vi "Polarizer_calib_find_zero_6.vi"(2 "Tolerance":dbl=0.1, 3 "Find Zero":bool, 6 "Medir pasos\n por vuelta":bool, 7 "Angulo \ndeseado":dbl, 8 "Argumento":string="50", 9 "Número de motor":string="1", 10 "Pasos por \nvuelta":dbl=757.0, 11 "Go to angle":bool) -> ()   [LabVIEW 2013]
uses:
  <vilib>/Analysis/baseanly.llb/Mean (DBL).vi
  <vilib>/Utility/file.llb/Write To Spreadsheet File (DBL).vi
  <vilib>/regexp/Match Regular Expression.xnode
  <vilib>/Analysis/NI_AALBase.lvlib
panel:
  out "Find Zero S2":bool
  out "Error":dbl format="%#_4g"
  out "Min value":dbl
  out "Cero absoluto":dbl
  in  "Find Zero 2":bool
  in  "Pasos por vuelta para cada motor\nM1(757)        M2(661)      M3(744)      M4(751)":dbl[](array[numeric])=[757.0, 661.0, 744.0, 751.0]
  out "Angulo \nfinal":dbl
  out "Angulo por\npaso":dbl
  in  "Restart \n Arduino":bool
  in  "Stop VI":bool
  in  "wait until completion? (T)":bool=TRUE
  in  "Boolean 2":bool
  in  "Set speed":bool
  in  "Current Step":bool
  in  "Set Zero":bool
  in  "Shutter off":bool
  in  "Shutter on":bool
  in  "Stop":bool
  in  "Go to step":bool
  in  "Constant speed":bool
  in  "Comando":string
  in  "x":bool
  out "x > y?":bool
  in  "x1":bool
  out "Array":string[](array[string])
  in  "Tab Control":enum32{"Live Picture", "ICImagingControl "}(tab)
  out "Live Picture":picture
  in  "ICImagingControl 2":refnum<k7>(container)
  out "nearest integer value":dbl
  out "Terminal output":string
  in  "Directorio scripts ArduinoStepper.py":path=path "C:/Users/franjas/Documents/rutinas-calibracion-slm"
  out "Comando que está siendo enviado a python":string
  in  "Zero_bol":bool
  out "Current Value":dbl format="%0.2f"
  in  "Save history data":bool
  out "Waveform Chart":dbl(graph)
  out "Found minimum":bool=TRUE
  out "i old":i32
  out "Waveform Chart 2":dbl(graph)
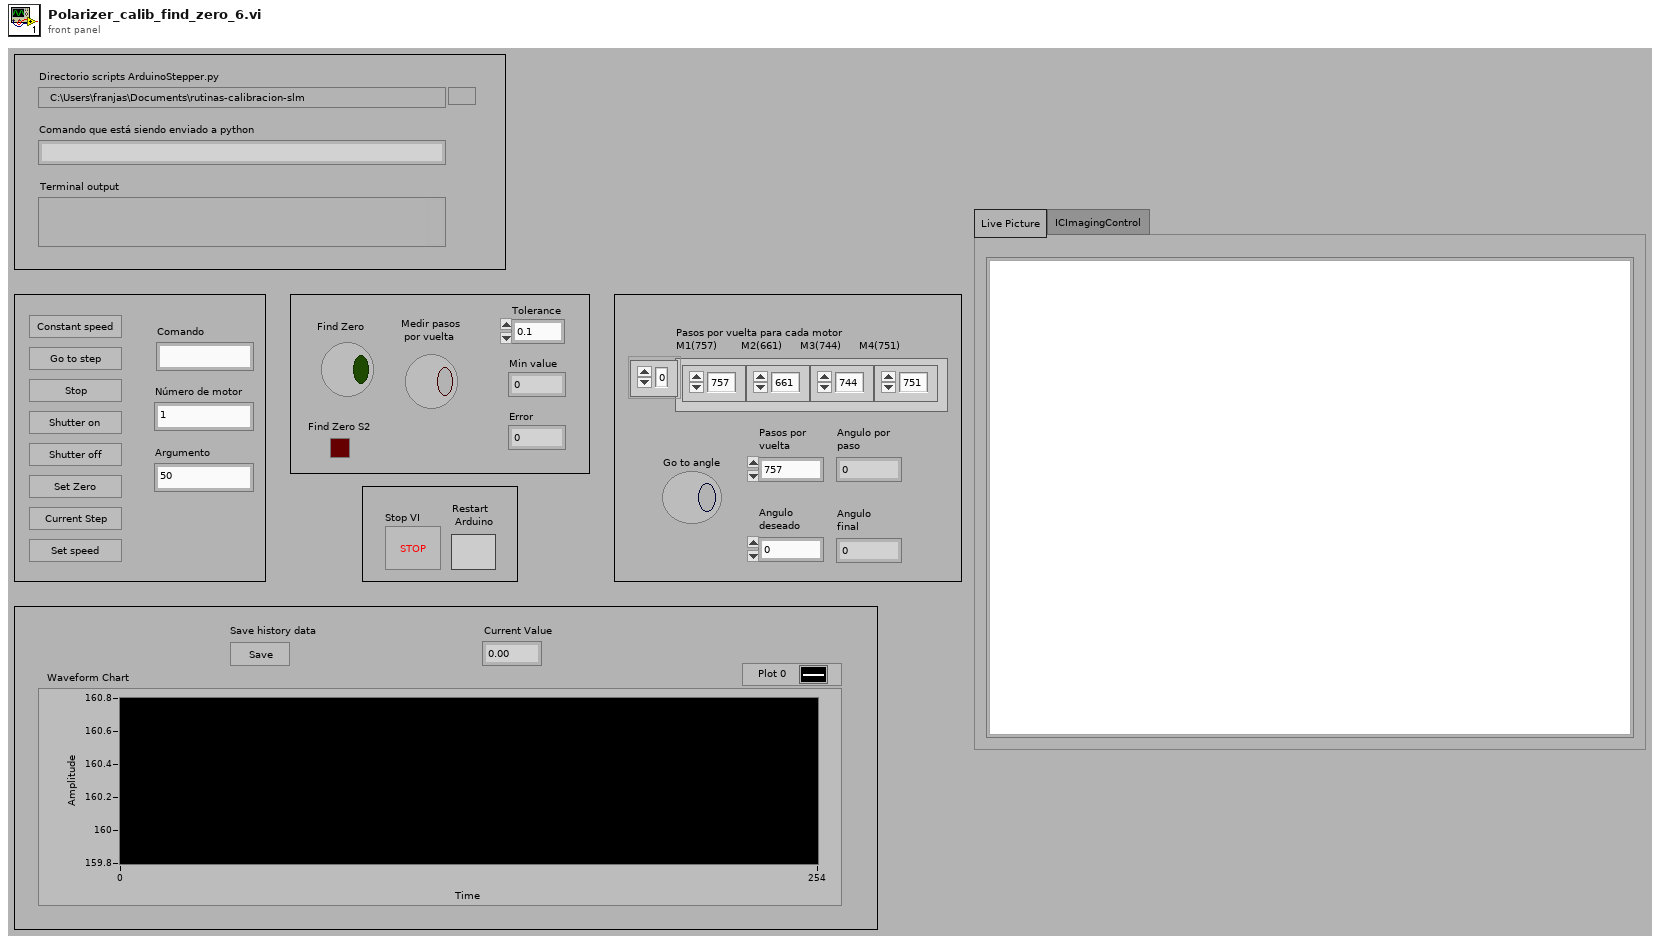
[diagram p1: front panel]
types:
  T1 = typedef "imagedata.ctl" = cluster{"image type":i32, "image depth":i32, "image":u8[], "mask":u8[], "colors":u32[], "Rectangle":cluster{"left":i16, "top":i16, "right":i16, "bottom":i16}}
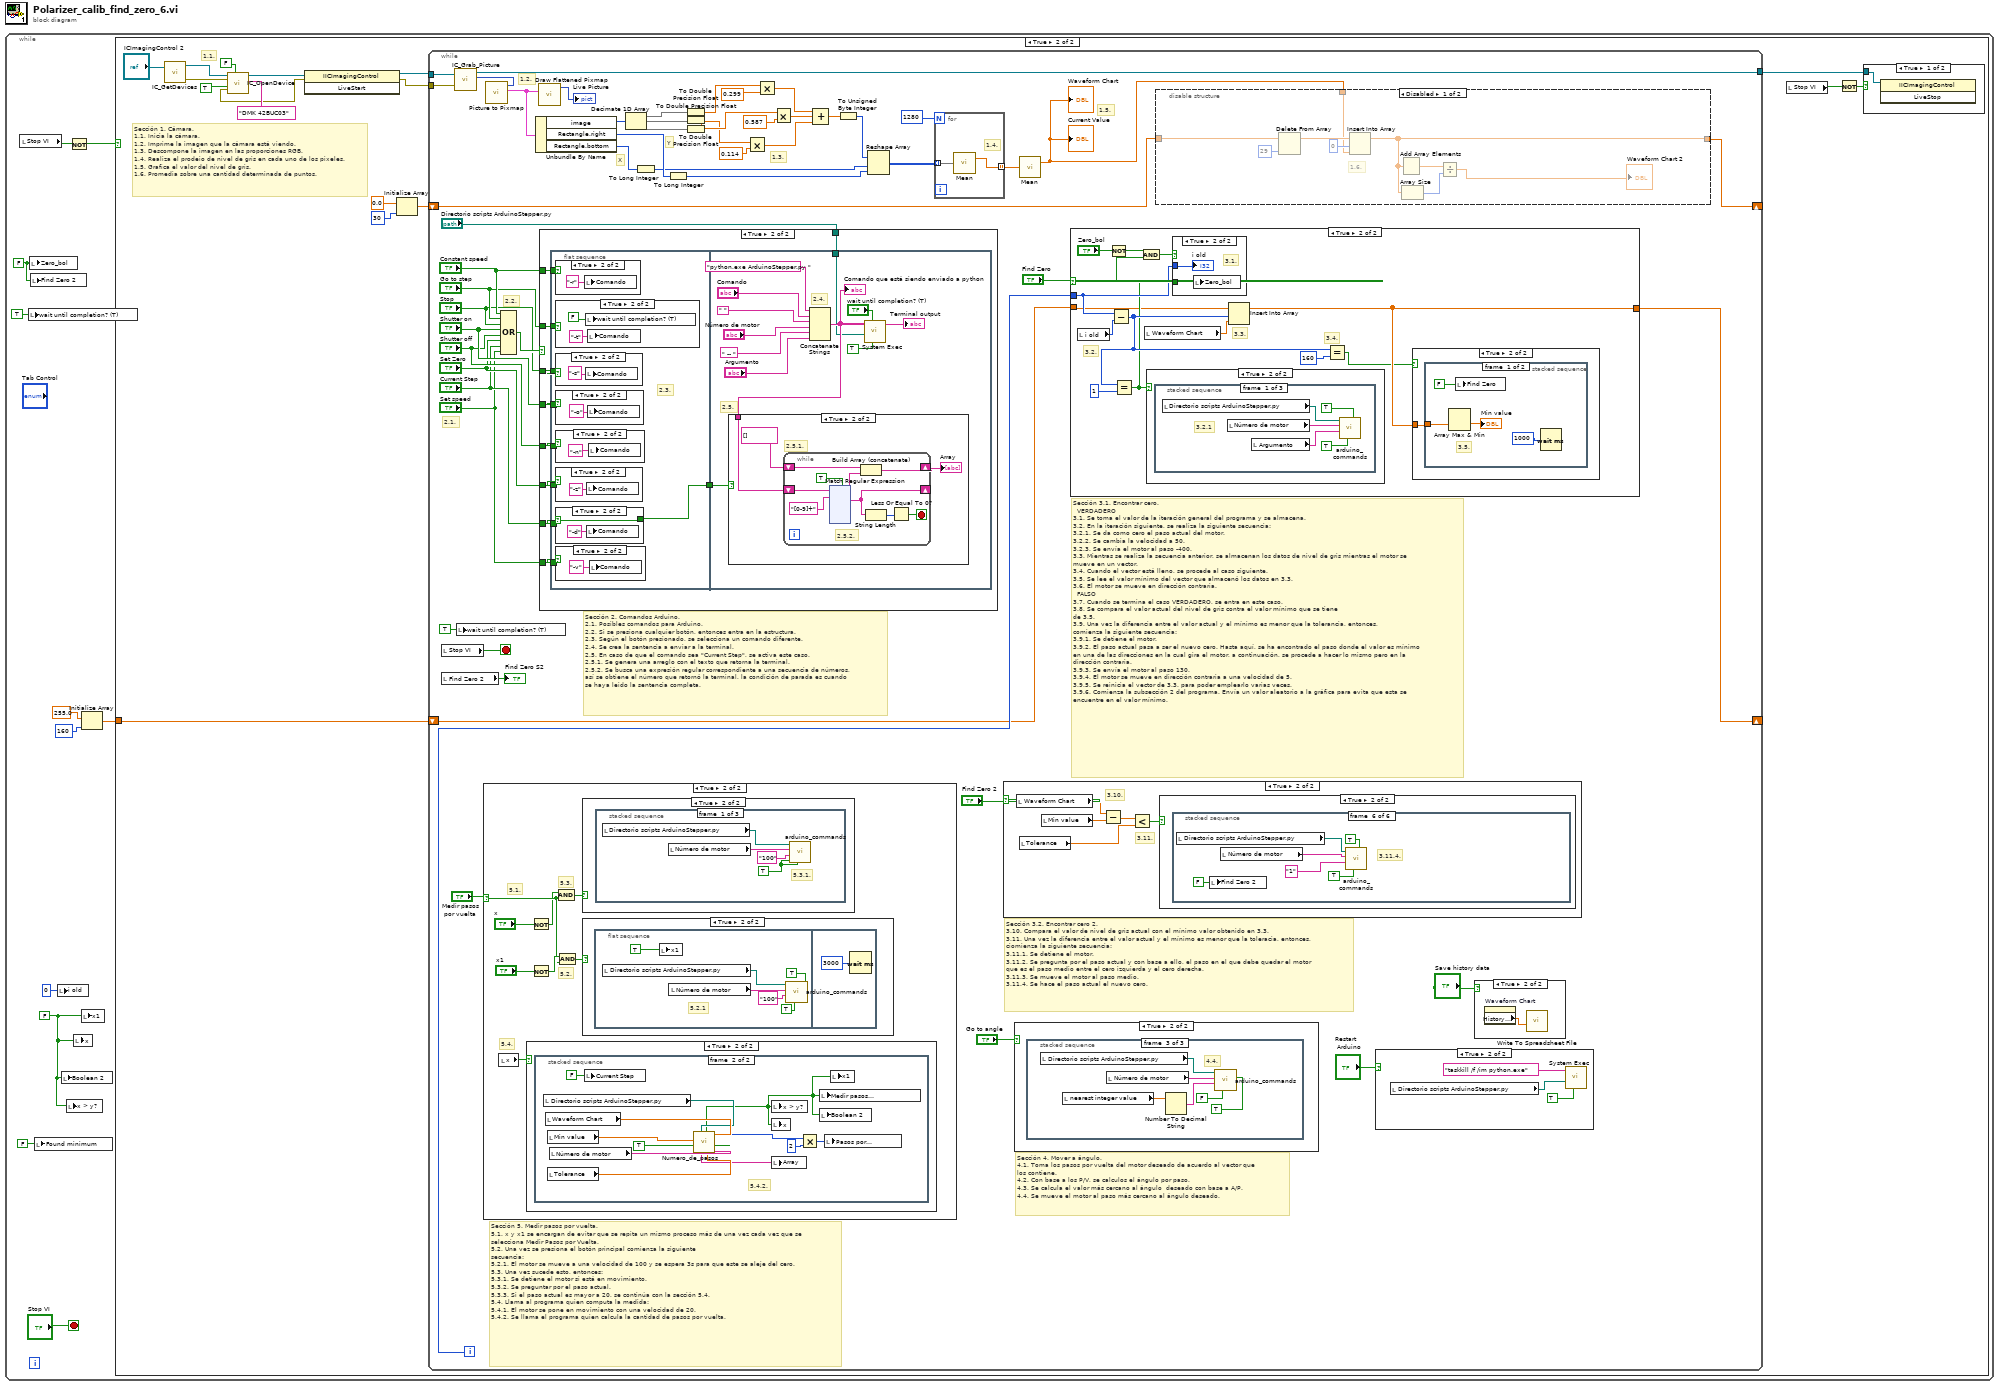
[diagram p0: block diagram]
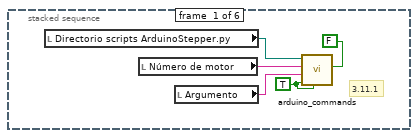
[diagram p6: hidden frame]
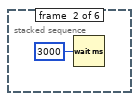
[diagram p7: hidden frame]
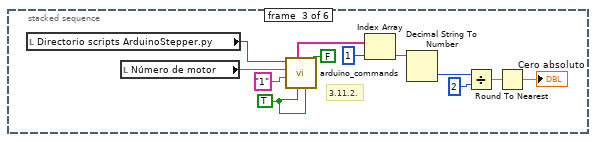
[diagram p8: hidden frame]
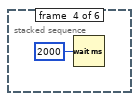
[diagram p9: hidden frame]
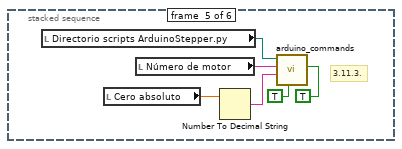
[diagram p10: hidden frame]
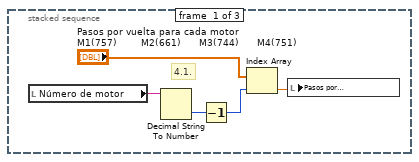
[diagram p13: hidden frame]
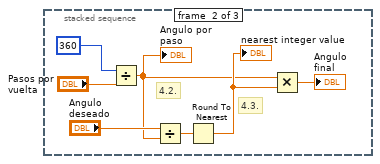
[diagram p14: hidden frame]
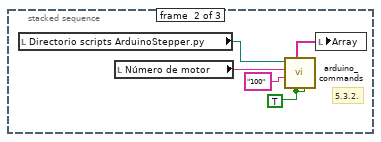
[diagram p17: hidden frame]
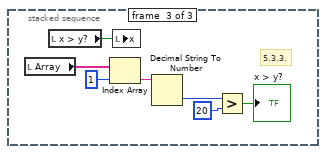
[diagram p18: hidden frame]
diagram:
  n1 = while {
    stop <- "Stop VI" stop-if-true
    w3 = FALSE ("Boolean")
    w1 = FALSE ("Zero_bol")
    n2 = local read "Stop VI"() -> (w5:bool)
    n3 = local write "wait until completion? (T)"(TRUE ("wait until completion? (T)")) -> ()
    n4 = local write "Zero_bol"(w1) -> ()
    n5 = local write "Find Zero 2"(w1) -> ()
    n6 = local write "Found minimum"(FALSE ("Found minimum")) -> ()
    n7 = local write "i old"(0 ("i old")) -> ()
    n8 = local write "Boolean 2"(w3) -> ()
    n9 = local write "x > y?"(w3) -> ()
    n10 = Not(x=w5) -> (.not. x?=w6:bool)
    n11 = local write "x"(w3) -> ()
    n12 = Initialize Array(255.0 ("element"), 160 ("dimension size")) -> (w9:dbl[])
    n13 = local write "x1"(w3) -> ()
    n14 = case shown="True" w6 {
      tunnel: w9 -> [_ w16]
      frame False {
      }
      frame True {
        # "Sección 1. Cámara. \n1.1. Inicia la cámara.\n1.2. Imprime la imagen que la cámara está viendo.\n1.3. Descompone la imagen en las proporciones RGB.\n1.4. Realiza el prodeio de nivel de gris en cada uno de los pixeles.\n1.5. Grafica el valor del nivel de gris.\n1.6. Promedia sobre una cantidad determinada de puntos."
        # "1.1."
        n15 = call <userlib>:"IC_GetDevices.vi"("ICImagingControl In"="ICImagingControl 2") -> ("ICImagingControl Out"=w26:refnum<k7>, "Error Out"=w22:errorcluster)  [unwired: 1 in, 1 out]
        n16 = call <userlib>:"IC_OpenDevice.vi"("Color"=FALSE, "Error In (no error)"=w22, "Live"=TRUE, "Device"="DMK 42BUC03", "ICImagingControl In"=w26) -> ("ICImagingControl Out"=w23:refnum<k7>, "Error Out"=w21:errorcluster)  [unwired: 1 in, 4 out]
        n17 = invoke class="IICImagingControl" method="LiveStart"(reference=w23, error in=w21) -> (reference out=w15:refnum<k7>, error out=w20:errorcluster)  [unwired: 1 in, 1 out]
        n18 = Initialize Array "Initialize Array"(0.0 ("element"), 30 ("dimension size")) -> (w14:dbl[])
        n19 = while {
          tunnel: w15 -> [w78]
          tunnel: w20 -> [w48]
          tunnel: [w79] -> w19
          shift-right: [w29] -> _
          shift-left: w14 -> [w60]
          shift-right: [w30] -> _
          shift-left: w16 -> [w58]
          i -> [w59]
          stop <- w54 stop-if-true
          # "Sección 5. Medir pasos por vuelta.\n5.1. x y x1 se encargan de evitar que se repita un mismo proceso más de una vez cada vez que se \nselecciona Medir Pasos por Vuelta. \n5.2. Una vez se presiona el botón principal comienza la siguiente\nsecuencia:\n5.2.1. El motor se mueve a una velocidad de 100 y se espera 3s para que este se aleje del cero.\n5.3. Una vez sucede esto, entonces:\n5.3.1. Se detiene el motor si está en movimiento.\n5.3.2. Se preguntar por el paso actual.\n5.3.3. Si el paso actual es mayor a 20, se continúa con la sección 5.4.\n5.4. Llama al programa quien computa la medida:\n5.4.1. El motor se pone en movimiento con una velocidad de 20.\n5.4.2. Se llama el programa quien calcula la cantidad de pasos por vuelta."
          # "Sección 3.2. Encontrar cero 2.\n3.10. Compara el valor de nivel de gris actual con el mínimo valor obtenido en 3.3.\n3.11. Una vez la diferencia entre el valor actual y el mínimo es menor que la toleracia, entonces, \nciomienza la siguiente secuencia:\n3.11.1. Se detiene el motor.\n3.11.2. Se pregunta por el paso actual y con base a ello, el paso en el que debe quedar el motor\nque es el paso medio entre el cero izquierda y el cero derecha.\n3.11.3. Se mueve el motor al paso medio.\n3.11.4. Se hace el paso actual el nuevo cero."
          # "Sección 3.1. Encontrar cero.\n  VERDADERO\n3.1. Se toma el valor de la iteración general del programa y se almacena.\n3.2. En la iteración siguiente, se realiza la siguiente secuencia:\n3.2.1. Se da como cero el paso actual del motor.\n3.2.2. Se cambia la velocidad a 50.\n3.2.3. Se envía el motor al paso -400.\n3.3. Mientras se realiza la secuencia anterior, se almacenan los datos de nivel de gris mientras el motor se \nmueve en un vector.\n3.4. Cuando el vector está lleno, se procede al caso siguiente.\n3.5. Se lee el valor mínimo del vector que almacenó los datos en 3.3. \n3.6. El motor se mueve en dirección contraria.\n  FALSO\n3.7. Cuando se termina el caso VERDADERO, se entra en este caso.\n3.8. Se compara el valor actual del nivel de gris contra el valor mínimo que se tiene\nde 3.5.\n3.9. Una vez la diferencia entre el valor actual y el mínimo es menor que la tolerancia, entonces, \ncomienza la siguiente secuencia:\n3.9.1. Se detiene el motor.\n3.9.2. El paso actual pasa a ser el nuevo cero. Hasta aquí, se ha encontrado el paso donde el valor es mínimo\nen una de las direcciones en la cual gira el motor, a continuación, se procede a hacer lo mismo pero en la \ndirección contraria. \n3.9.3. Se envía el motor al paso 130.\n3.9.4. El motor se mueve en dirección contraria a una velocidad de 5.\n3.9.5. Se reinicia el vector de 3.3. para poder emplearlo varias veces.\n3.9.6. Comienza la subsección 2 del programa. Envía un valor aleatorio a la gráfica para evita que esta se \nencuentre en el valor mínimo."
          # "Sección 4. Mover a ángulo.\n4.1. Toma los pasos por vuelta del motor deseado de acuerdo al vector que\nlos contiene.\n4.2. Con base a los P/V, se calculos el ángulo por paso.\n4.3. Se calcula el valor más cercano al ángulo  deseado con base a A/P.\n4.4. Se mueve el motor al paso más cercano al ángulo deseado."
          # "2.2."
          # "2.1."
          # "Sección 2. Comandos Arduino.\n2.1. Posibles comandos para Arduino.\n2.2. Si se presiona cualquier botón, entonces entra en la estructura.\n2.3. Según el botón presionado, se selecciona un comando diferente.\n2.4. Se crea la sentencia a enviar a la terminal.\n2.5. En caso de que el comando sea \"Current Step\", se activa este caso.\n2.5.1. Se genera una arreglo con el texto que retorna la terminal.\n2.5.2. Se busca una expresión regular correspondiente a una secuencia de números,\nasí se obtiene el número que retornó la terminal, la condición de parada es cuando\nse haya leido la sentencia completa."
          # "1.5."
          # "1.3."
          # "1.2."
          # "Y"
          # "X"
          n20 = local read "Stop VI"() -> (w54:bool)
          n21 = local read "Find Zero 2"() -> (→"Find Zero S2":bool)
          n22 = call <userlib>:"IC_Grab_Picture.vi"("ICImagingControl In"=w78, "Error In (no error)"=w48) -> ("ICImagingControl Out"=w79:refnum<k7>, "Picture Out"=w81:picture)  [unwired: 2 out]
          n23 = local write "wait until completion? (T)"(TRUE ("wait until completion? (T)")) -> ()
          n24 = case shown="True" "Medir pasos\n por vuelta" {
            selector: "Medir pasos\n por vuelta" -> [_ w143]
            frame False {
            }
            frame True {
              # "5.4."
              # "5.3."
              # "5.2."
              # "5.1."
              n25 = local read "x"() -> (w140:bool)
              n26 = case shown="True" w140 {
                frame False {
                }
                frame True {
                  n27 = stacked-sequence {
                    frame #0 {
                      n28 = Not(x="Boolean 2") -> (.not. x?=w171:bool)
                      n29 = case shown="True" w171 {
                        frame False {
                        }
                        frame True {
                          w174 = TRUE ("Constant speed")
                          # "5.4.1."
                          n30 = local read "Directorio scripts ArduinoStepper.py"() -> (w176:path)
                          n31 = local read "Número de motor"() -> (w177:string)
                          n32 = local write "Boolean 2"(w174) -> ()
                          n33 = call "arduino_commands.vi"("Constant speed"=w174, "Wait until completion? (T)"=FALSE ("wait until completion? (T)"), "Argumento"="20", "Número de motor"=w177, "Directorio scripts ArduinoStepper.py"=w176) -> ()  [unwired: 6 in, 1 out]
                        }
                      }
                    }
                    frame #1 {
                      # "5.4.2."
                      n34 = local read "Directorio scripts ArduinoStepper.py"() -> (w187:path)
                      n35 = local read "Waveform Chart"() -> (w189:dbl)
                      n36 = local read "Min value"() -> (w188:dbl)
                      n37 = local read "Tolerance"() -> (w185:dbl)
                      n38 = local read "Número de motor"() -> (w186:string)
                      n39 = local write "Current Step"(FALSE ("Current Step")) -> ()
                      n40 = call "Numero_de_pasos.vi"("Tolerance"=w185, "Directorio scripts ArduinoStepper.py"=w187, "Número de motor"=w186, "Medir pasos por\nvuelta"=TRUE ("Medir pasos por\nvuelta"), "Minimo"=w188, "Valor actual"=w189) -> ("Media vuelta"=w182:i32, "Proceso en \nejecución"=w179:bool, "Array"=w178:string[])  [unwired: 3 in]
                      n41 = local write "x > y?"(w179) -> ()
                      n42 = local write "x"(w179) -> ()
                      n43 = local write "Array"(w178) -> ()
                      n44 = Multiply(x=w182, y=2) -> (x*y=w180:i32)
                      n45 = local write "Medir pasos\n por vuelta"(w179) -> ()
                      n46 = local write "Boolean 2"(w179) -> ()
                      n47 = local write "Pasos por \nvuelta"(w180) -> ()
                      n48 = local write "x1"(w179) -> ()
                    }
                  }
                }
              }
              n49 = Not(x="x") -> (.not. x?=w141:bool)
              n50 = Not(x="x1") -> (.not. x?=w147:bool)
              n51 = And(x=w141, y=w143) -> (x .and. y?=w144:bool)
              n52 = And(x=w147, y=w143) -> (x .and. y?=w145:bool)
              n53 = case shown="True" w144 {
                frame False {
                }
                frame True {
                  n54 = stacked-sequence {
                    frame #0 {
                      w148 = TRUE ("Constant speed")
                      # "5.3.1."
                      n55 = local read "Directorio scripts ArduinoStepper.py"() -> (w150:path)
                      n56 = local read "Número de motor"() -> (w151:string)
                      n57 = call "arduino_commands.vi"("Wait until completion? (T)"=w148, "Stop"=w148, "Argumento"="100", "Número de motor"=w151, "Directorio scripts ArduinoStepper.py"=w150) -> ()  [unwired: 6 in, 1 out]
                    }
                    frame #1 {
                      w152 = TRUE ("wait until completion? (T)")
                      # "5.3.2."
                      n58 = local read "Directorio scripts ArduinoStepper.py"() -> (w155:path)
                      n59 = local read "Número de motor"() -> (w156:string)
                      n60 = call "arduino_commands.vi"("Current Step"=w152, "Wait until completion? (T)"=w152, "Argumento"="100", "Número de motor"=w156, "Directorio scripts ArduinoStepper.py"=w155) -> ("Retorno terminal"=w153:string[])  [unwired: 6 in]
                      n61 = local write "Array"(w153) -> ()
                    }
                    frame #2 {
                      # "5.3.3."
                      n62 = local read "Array"() -> (w161:string[])
                      n63 = local read "x > y?"() -> (w159:bool)
                      n64 = Index Array(array=w161, index=1) -> (element=w160:string)
                      n65 = local write "x"(w159) -> ()
                      n66 = Decimal String To Number(string=w160) -> (number=w162:i32)  [unwired: 2 in, 1 out]
                      n67 = Greater?(x=w162, y=20) -> (0:→"x > y?":bool)
                    }
                  }
                }
              }
              n68 = case shown="True" w145 {
                frame False {
                }
                frame True {
                  n69 = flat-sequence {
                    frame #0 {
                      # "5.2.1"
                      n70 = local read "Directorio scripts ArduinoStepper.py"() -> (w168:path)
                      n71 = local write "x1"(TRUE ("Boolean")) -> ()
                      n72 = local read "Número de motor"() -> (w167:string)
                      n73 = call "arduino_commands.vi"("Constant speed"=TRUE, "Wait until completion? (T)"=TRUE ("wait until completion? (T)"), "Argumento"="100", "Número de motor"=w167, "Directorio scripts ArduinoStepper.py"=w168) -> ()  [unwired: 6 in, 1 out]
                    }
                    frame #1 {
                      n74 = Wait (ms)(milliseconds to wait=u32 3000) -> ()  [unwired: 1 out]
                    }
                  }
                }
              }
            }
          }
          n75 = call <vilib>:"Picture to Pixmap.vi"("picture"=w81) -> ("image data"=w71:T1)  [unwired: 9 in, 1 out]
          n76 = Compound Arithmetic op=OR("Constant speed", "Go to step", "Stop", "Shutter on", "Shutter off", "Set Zero", "Current Step", "Set speed") -> (w42:bool)
          n77 = Unbundle By Name(w71) -> ("image"=w47:u8[], "Rectangle.right"=w75:i16, "Rectangle.bottom"=w73:i16)
          n78 = call <vilib>:"Draw Flattened Pixmap.vi"("image data"=w71) -> ("new picture"=→"Live Picture":picture)  [unwired: 8 in]
          n79 = case shown="True" w42 {
            tunnel: "Constant speed" -> [_ w292]
            tunnel: "Go to step" -> [_ w291]
            tunnel: "Stop" -> [_ w290]
            tunnel: "Shutter on" -> [_ w289]
            tunnel: "Shutter off" -> [_ w288]
            tunnel: "Set Zero" -> [_ w287]
            tunnel: "Current Step" -> [_ w286]
            tunnel: "Set speed" -> [_ w285]
            tunnel: "Directorio scripts ArduinoStepper.py" -> [_ w283]
            frame False {
            }
            frame True {
              n80 = flat-sequence {
                tunnel: w292 -> [w301]
                tunnel: w291 -> [w300]
                tunnel: w290 -> [w299]
                tunnel: w289 -> [w298]
                tunnel: w288 -> [w297]
                tunnel: w287 -> [w296]
                tunnel: w286 -> [w295]
                tunnel: w285 -> [w294]
                tunnel: [w293] -> w284
                tunnel: w284 -> [w315]
                tunnel: w283 -> [w314]
                frame #0 {
                  # "2.3."
                  n81 = case shown="True" w301 {
                    frame False {
                    }
                    frame True {
                      n82 = local write "Comando"("-r" ("Comando")) -> ()
                    }
                  }
                  n83 = case shown="True" w300 {
                    frame False {
                    }
                    frame True {
                      n84 = local write "wait until completion? (T)"(FALSE ("wait until completion? (T)")) -> ()
                      n85 = local write "Comando"("-t" ("Comando")) -> ()
                    }
                  }
                  n86 = case shown="True" w299 {
                    frame False {
                    }
                    frame True {
                      n87 = local write "Comando"("-s" ("Comando")) -> ()
                    }
                  }
                  n88 = case shown="True" w298 {
                    frame False {
                    }
                    frame True {
                      n89 = local write "Comando"("-o" ("Comando")) -> ()
                    }
                  }
                  n90 = case shown="True" w297 {
                    frame False {
                    }
                    frame True {
                      n91 = local write "Comando"("-n" ("Comando")) -> ()
                    }
                  }
                  n92 = case shown="True" w296 {
                    frame False {
                    }
                    frame True {
                      n93 = local write "Comando"("-z" ("Comando")) -> ()
                    }
                  }
                  n94 = case shown="True" w295 {
                    selector: w295 -> [w303 w304]
                    tunnel: [w303 w304] -> w293
                    frame False {
                    }
                    frame True {
                      n95 = local write "Comando"("-d" ("Comando")) -> ()
                    }
                  }
                  n96 = case shown="True" w294 {
                    frame False {
                    }
                    frame True {
                      n97 = local write "Comando"("-v" ("Comando")) -> ()
                    }
                  }
                }
                frame #1 {
                  # "2.5."
                  # "2.4."
                  n98 = Concatenate Strings("python.exe ArduinoStepper.py ", "Comando", " " ("string"), "Número de motor", " -- ", "Argumento") -> (w317:string)
                  "Comando que está siendo enviado a python" <- w317
                  n99 = call <vilib>:"System Exec.vi"("run minimized? (F)"=TRUE, "wait until completion? (T)"="wait until completion? (T)", "working directory"=w314, "command line"=w317) -> ("standard output"=w324:string)  [unwired: 4 in, 3 out]
                  "Terminal output" <- w324
                  n100 = case shown="True" w315 {
                    tunnel: w324 -> [_ w327]
                    frame False {
                    }
                    frame True {
                      # "2.5.1."
                      n101 = while {
                        shift-right: [w335] -> _
                        shift-left: w327 -> [w329]
                        shift-right: [w333] -> w326
                        shift-left: string[] [] -> [w331]
                        stop <- w328 stop-if-true
                        # "2.5.2."
                        n102 = xnode "Match Regular Expression"("input string"=w329, "regular expression"="[0-9]+", "multiline? (F)"=TRUE) -> ("whole match"=w332:string, "after match"=w335:string)  [unwired: 3 in, 5 out]
                        n103 = Build Array (concatenate)(w331, w332) -> (w333:string[])
                        n104 = String Length(string=w335) -> (length=w334:i32)
                        n105 = Less Or Equal To 0?(x=w334) -> (x <= 0?=w328:bool)
                      }
                      "Array" <- w326
                    }
                  }
                }
              }
            }
          }
          n106 = Decimate 1D Array(w47) -> (w61:u8[], w46:u8[], w45:u8[])
          n107 = To Long Integer(number=w73) -> (32bit integer=w72:i32)
          n108 = To Long Integer(number=w75) -> (32bit integer=w74:i32)
          n109 = To Double Precision Float(number=w61) -> (double precision float=w69:dbl[])
          n110 = To Double Precision Float(number=w46) -> (double precision float=w68:dbl[])
          n111 = To Double Precision Float(number=w45) -> (double precision float=w67:dbl[])
          n112 = Multiply(x=w67, y=0.114) -> (x*y=w62:dbl[])
          n113 = Multiply(x=w69, y=0.299) -> (x*y=w64:dbl[])
          n114 = Multiply(x=w68, y=0.587) -> (x*y=w63:dbl[])
          n115 = Compound Arithmetic op=ADD(w64, w63, w62) -> (w43:dbl[])
          n116 = To Unsigned Byte Integer(number=w43) -> (unsigned 8bit integer=w76:u8[])
          n117 = Reshape Array(w76, w72, w74) -> (w70:u8[][])
          n118 = for {
            N: 1280 -> [_]
            tunnel: [w455] -> w80 mode=indexing
            tunnel: w70 -> [w454] mode=indexing
            # "1.4."
            n119 = call-poly <vilib>:"Mean.vi"("X"=w454) -> ("mean"=w455:dbl)  [unwired: 1 out]
          }
          n120 = case shown="True" "Find Zero 2" {
            frame False {
            }
            frame True {
              # "3.11."
              # "3.10."
              n121 = local read "Waveform Chart"() -> (w87:dbl)
              n122 = local read "Tolerance"() -> (w85:dbl)
              n123 = local read "Min value"() -> (w86:dbl)
              n124 = Subtract(x=w87, y=w86) -> (x-y=w84:dbl)
              n125 = Less?(x=w84, y=w85) -> (x < y?=w83:bool)
              n126 = case shown="True" w83 {
                frame False {
                }
                frame True {
                  n127 = stacked-sequence {
                    frame #0 {
                      w88 = TRUE ("Stop")
                      # "3.11.1"
                      n128 = local read "Directorio scripts ArduinoStepper.py"() -> (w90:path)
                      n129 = local read "Número de motor"() -> (w91:string)
                      n130 = local read "Argumento"() -> (w92:string)
                      n131 = call "arduino_commands.vi"("Go to step"=FALSE, "Wait until completion? (T)"=w88, "Stop"=w88, "Argumento"=w92, "Número de motor"=w91, "Directorio scripts ArduinoStepper.py"=w90) -> ()  [unwired: 5 in, 1 out]
                    }
                    frame #1 {
                      n132 = Wait (ms)(milliseconds to wait=u32 3000) -> ()  [unwired: 1 out]
                    }
                    frame #2 {
                      w101 = TRUE ("Constant speed")
                      # "3.11.2."
                      n133 = local read "Directorio scripts ArduinoStepper.py"() -> (w99:path)
                      n134 = local read "Número de motor"() -> (w100:string)
                      n135 = call "arduino_commands.vi"("Go to step"=FALSE, "Current Step"=w101, "Wait until completion? (T)"=w101, "Argumento"="1", "Número de motor"=w100, "Directorio scripts ArduinoStepper.py"=w99) -> ("Retorno terminal"=w104:string[])  [unwired: 5 in]
                      n136 = Index Array(array=w104, index=1) -> (element=w103:string)
                      n137 = Decimal String To Number(string=w103) -> (number=w97:i32)  [unwired: 2 in, 1 out]
                      n138 = Divide(x=w97, y=2) -> (x/y=w96:dbl)
                      n139 = Round To Nearest(number=w96) -> (nearest integer value=→"Cero absoluto":dbl)
                    }
                    frame #3 {
                      n140 = Wait (ms)(milliseconds to wait=u32 2000) -> ()  [unwired: 1 out]
                    }
                    frame #4 {
                      # "3.11.3."
                      n141 = local read "Directorio scripts ArduinoStepper.py"() -> (w110:path)
                      n142 = local read "Cero absoluto"() -> (w109:dbl)
                      n143 = local read "Número de motor"() -> (w111:string)
                      n144 = Number To Decimal String(number=w109) -> (decimal integer string=w112:string)  [unwired: 1 in]
                      n145 = call "arduino_commands.vi"("Go to step"=TRUE, "Wait until completion? (T)"=TRUE ("wait until completion? (T)"), "Argumento"=w112, "Número de motor"=w111, "Directorio scripts ArduinoStepper.py"=w110) -> ()  [unwired: 6 in, 1 out]
                    }
                    frame #5 {
                      # "3.11.4."
                      n146 = local read "Directorio scripts ArduinoStepper.py"() -> (w117:path)
                      n147 = local write "Find Zero 2"(FALSE ("Find Zero 2")) -> ()
                      n148 = local read "Número de motor"() -> (w116:string)
                      n149 = call "arduino_commands.vi"("Set zero"=TRUE, "Wait until completion? (T)"=TRUE, "Argumento"="1", "Número de motor"=w116, "Directorio scripts ArduinoStepper.py"=w117) -> ()  [unwired: 6 in, 1 out]
                    }
                  }
                }
              }
            }
          }
          n150 = case shown="True" "Go to angle" {
            frame False {
            }
            frame True {
              n151 = stacked-sequence {
                frame #0 {
                  # "4.1."
                  n152 = local read "Número de motor"() -> (w125:string)
                  n153 = Decimal String To Number(string=w125) -> (number=w126:i32)  [unwired: 2 in, 1 out]
                  n154 = Decrement(x=w126) -> (x-1=w123:i32)
                  n155 = Index Array(array="Pasos por vuelta para cada motor\nM1(757)        M2(661)      M3(744)      M4(751)", index=w123) -> (element=w124:dbl)
                  n156 = local write "Pasos por \nvuelta"(w124) -> ()
                }
                frame #1 {
                  # "4.3."
                  # "4.2."
                  n157 = Divide(x=360, y="Pasos por \nvuelta") -> (x/y=w128:dbl)
                  "Angulo por\npaso" <- w128
                  n158 = Divide(x="Angulo \ndeseado", y=w128) -> (x/y=w130:dbl)
                  n159 = Round To Nearest(number=w130) -> (nearest integer value=w129:dbl)
                  "nearest integer value" <- w129
                  n160 = Multiply(x=w128, y=w129) -> (x*y=→"Angulo \nfinal":dbl)
                }
                frame #2 {
                  # "4.4."
                  n161 = local read "Directorio scripts ArduinoStepper.py"() -> (w139:path)
                  n162 = local read "nearest integer value"() -> (w135:dbl)
                  n163 = local read "Número de motor"() -> (w138:string)
                  n164 = Number To Decimal String(number=w135) -> (decimal integer string=w136:string)  [unwired: 1 in]
                  n165 = call "arduino_commands.vi"("Go to step"=TRUE, "Wait until completion? (T)"=FALSE ("wait until completion? (T)"), "Argumento"=w136, "Número de motor"=w138, "Directorio scripts ArduinoStepper.py"=w139) -> ()  [unwired: 6 in, 1 out]
                }
              }
            }
          }
          n166 = call-poly <vilib>:"Mean.vi"("X"=w80) -> ("mean"=w56:dbl)  [unwired: 1 out]
          "Waveform Chart" <- w56
          "Current Value" <- w56
          n167 = case shown="True" "Find Zero" {
            selector: "Find Zero" -> [_ w249]
            tunnel: w58 -> [w200 w243]
            tunnel: w59 -> [_ w245]
            tunnel: [w199 w252] -> w30
            frame False {
              # "3.7."
              n168 = local read "Found minimum"() -> (w201:bool)
              n169 = case shown="True" w201 {
                tunnel: [w202 w205] -> w199
                tunnel: w200 -> [w202 w204]
                frame False {
                }
                frame True {
                  # "3.9."
                  # "3.8."
                  n170 = local read "Waveform Chart"() -> (w207:dbl)
                  n171 = local read "Min value"() -> (w209:dbl)
                  n172 = Subtract(x=w207, y=w209) -> (x-y=w203:dbl)
                  "Error" <- w203
                  n173 = Less?(x=w203, y="Tolerance") -> (x < y?=w208:bool)
                  n174 = case shown="True" w208 {
                    tunnel: [w210 w212] -> w205
                    tunnel: w204 -> [w210 w211]
                    frame False {
                    }
                    frame True {
                      n175 = stacked-sequence {
                        tunnel: [_ _ _ _ _ w234 _] -> w212
                        tunnel: w211 -> [_ _ _ _ _ w233 _]
                        frame #0 {
                          w213 = TRUE ("Stop")
                          # "3.9.1."
                          n176 = local read "Directorio scripts ArduinoStepper.py"() -> (w216:path)
                          n177 = local read "Número de motor"() -> (w215:string)
                          n178 = local read "Argumento"() -> (w214:string)
                          n179 = call "arduino_commands.vi"("Wait until completion? (T)"=w213, "Stop"=w213, "Argumento"=w214, "Número de motor"=w215, "Directorio scripts ArduinoStepper.py"=w216) -> ()  [unwired: 6 in, 1 out]
                        }
                        frame #1 {
                          w217 = TRUE ("wait until completion? (T)")
                          # "3.9.2."
                          n180 = local read "Directorio scripts ArduinoStepper.py"() -> (w222:path)
                          n181 = local write "Zero_bol"(FALSE ("zero_bol")) -> ()
                          n182 = local write "Found minimum"(FALSE ("Found minimum")) -> ()
                          n183 = local read "Número de motor"() -> (w221:string)
                          n184 = local read "Argumento"() -> (w220:string)
                          n185 = call "arduino_commands.vi"("Set zero"=w217, "Wait until completion? (T)"=w217, "Argumento"=w220, "Número de motor"=w221, "Directorio scripts ArduinoStepper.py"=w222) -> ()  [unwired: 6 in, 1 out]
                        }
                        frame #2 {
                          w223 = TRUE ("wait until completion? (T)")
                          # "3.9.3."
                          n186 = local read "Directorio scripts ArduinoStepper.py"() -> (w227:path)
                          n187 = local read "Número de motor"() -> (w226:string)
                          n188 = Number To Decimal String(number=130 ("dimension size")) -> (decimal integer string=w224:string)  [unwired: 1 in]
                          n189 = call "arduino_commands.vi"("Go to step"=w223, "Wait until completion? (T)"=w223, "Argumento"=w224, "Número de motor"=w226, "Directorio scripts ArduinoStepper.py"=w227) -> ()  [unwired: 6 in, 1 out]
                        }
                        frame #3 {
                          w228 = TRUE ("Constant speed")
                          # "3.9.4."
                          n190 = local read "Directorio scripts ArduinoStepper.py"() -> (w231:path)
                          n191 = local read "Número de motor"() -> (w230:string)
                          n192 = call "arduino_commands.vi"("Constant speed"=w228, "Wait until completion? (T)"=w228, "Argumento"="-5", "Número de motor"=w230, "Directorio scripts ArduinoStepper.py"=w231) -> ()  [unwired: 6 in, 1 out]
                        }
                        frame #4 {
                          n193 = Wait (ms)(milliseconds to wait=u32 200) -> ()  [unwired: 1 out]
                        }
                        frame #5 {
                          # "3.9.5."
                          n194 = for {
                            N: 160 -> [_]
                            shift-right: [w236] -> w234
                            shift-left: w233 -> [w237]
                            i -> [w238]
                            n195 = Insert Into Array(array=w237, index=w238, new element=255.0 ("new element/subarray")) -> (w236:dbl[])
                          }
                        }
                        frame #6 {
                          # "3.9.6"
                          n196 = local write "Waveform Chart"(120.0 ("Waveform Chart")) -> ()
                          n197 = local write "Find Zero 2"(TRUE ("Find Zero 2")) -> ()
                        }
                      }
                    }
                  }
                }
              }
            }
            frame True {
              # "3.4."
              # "3.3."
              # "3.2."
              n198 = local read "i old"() -> (w248:i32)
              n199 = Not(x="Zero_bol") -> (.not. x?=w251:bool)
              n200 = Subtract(x=w245, y=w248) -> (x-y=w247:i32)
              n201 = Equal?(x=w247, y=1) -> (x = y?=w244:bool)
              n202 = And(x=w251, y=w249) -> (x .and. y?=w246:bool)
              n203 = local read "Waveform Chart"() -> (w255:dbl)
              n204 = case shown="True" w244 {
                frame False {
                }
                frame True {
                  n205 = stacked-sequence {
                    frame #0 {
                      # "3.2.1"
                      n206 = local read "Directorio scripts ArduinoStepper.py"() -> (w270:path)
                      n207 = local read "Número de motor"() -> (w269:string)
                      n208 = local read "Argumento"() -> (w268:string)
                      n209 = call "arduino_commands.vi"("Set zero"=TRUE, "Wait until completion? (T)"=TRUE ("wait until completion? (T)"), "Argumento"=w268, "Número de motor"=w269, "Directorio scripts ArduinoStepper.py"=w270) -> ()  [unwired: 6 in, 1 out]
                    }
                    frame #1 {
                      w272 = TRUE ("Set speed")
                      # "3.2.2."
                      n210 = local read "Directorio scripts ArduinoStepper.py"() -> (w273:path)
                      n211 = local read "Número de motor"() -> (w271:string)
                      n212 = call "arduino_commands_2.vi"("Número de motor"=w271, "Argumento"="50", "Directorio scripts ArduinoStepper.py"=w273, "wait until completion? (T)"=w272, "Set speed"=w272) -> ()  [unwired: 6 in]
                    }
                    frame #2 {
                      # "3.2.3."
                      n213 = local read "Directorio scripts ArduinoStepper.py"() -> (w280:path)
                      n214 = local read "Número de motor"() -> (w279:string)
                      n215 = Number To Decimal String(number=-400 ("dimension size")) -> (decimal integer string=w276:string)  [unwired: 1 in]
                      n216 = call "arduino_commands.vi"("Go to step"=TRUE, "Wait until completion? (T)"=FALSE ("wait until completion? (T)"), "Argumento"=w276, "Número de motor"=w279, "Directorio scripts ArduinoStepper.py"=w280) -> ()  [unwired: 6 in, 1 out]
                    }
                  }
                }
              }
              n217 = case shown="True" w246 {
                tunnel: w245 -> [_ w282]
                tunnel: w244 -> [_ w281]
                frame False {
                }
                frame True {
                  # "3.1."
                  n218 = local write "Zero_bol"(w281) -> ()
                  "i old" <- w282
                }
              }
              n219 = Insert Into Array(array=w243, index=w247, new element=w255) -> (w252:dbl[])
              n220 = Equal?(x=w247, y=160) -> (x = y?=w242:bool)
              n221 = case shown="True" w242 {
                tunnel: w252 -> [_ w256]
                frame False {
                }
                frame True {
                  n222 = stacked-sequence {
                    tunnel: w256 -> [w259 _]
                    frame #0 {
                      # "3.5."
                      n223 = Array Max & Min(array=w259) -> (min value=→"Min value":dbl)  [unwired: 3 out]
                      n224 = local write "Find Zero"(FALSE ("Zero")) -> ()
                      n225 = Wait (ms)(milliseconds to wait=u32 1000) -> ()  [unwired: 1 out]
                    }
                    frame #1 {
                      w261 = TRUE ("Constant speed")
                      # "3.6."
                      n226 = local read "Directorio scripts ArduinoStepper.py"() -> (w265:path)
                      n227 = local read "Número de motor"() -> (w264:string)
                      n228 = call "arduino_commands.vi"("Constant speed"=w261, "Wait until completion? (T)"=w261, "Argumento"="20", "Número de motor"=w264, "Directorio scripts ArduinoStepper.py"=w265) -> ()  [unwired: 6 in, 1 out]
                      "Found minimum" <- TRUE ("Found minimum")
                    }
                  }
                }
              }
            }
          }
          n229 = disable-structure shown="Disabled" {
            disable-tunnel: [w194 _] -> w29
            disable-tunnel: w60 -> [w193 _]
            disable-tunnel: w56 -> [w192 _]
            frame Disabled {
              # "1.6."
              n230 = Delete From Array "Delete From Array"(array=w193, index=29) -> (array with subset deleted=w198:dbl[])  [unwired: 1 in, 1 out]
              n231 = Insert Into Array "Insert Into Array"(array=w198, index=0, new element=w192) -> (w194:dbl[])
              n232 = Add Array Elements(numeric array=w194) -> (sum=w195:dbl)
              n233 = Array Size(array=w194) -> (size(s)=w191:i32)
              n234 = Divide(x=w195, y=w191) -> (x/y=→"Waveform Chart 2":dbl)
            }
            frame Enabled {
            }
          }
          n235 = case shown="True" "Restart \n Arduino" {
            frame False {
            }
            frame True {
              n236 = local read "Directorio scripts ArduinoStepper.py"() -> (w121:path)
              n237 = call <vilib>:"System Exec.vi"("run minimized? (F)"=TRUE, "working directory"=w121, "command line"="taskkill /f /im python.exe") -> ()  [unwired: 5 in, 4 out]
            }
          }
          n238 = case shown="True" "Save history data" {
            frame False {
            }
            frame True {
              n239 = property on="Waveform Chart" class="WFChart (strict)"() -> ("History Data"=w82:dbl[])  [unwired: 2 in, 2 out]
              n240 = call-poly <vilib>:"Write To Spreadsheet File.vi"("1D data"=w82) -> ()  [unwired: 7 in, 1 out]
            }
          }
        }
        n241 = local read "Stop VI"() -> (w13:bool)
        n242 = Not(x=w13) -> (.not. x?=w12:bool)
        n243 = case shown="True" w12 {
          tunnel: w19 -> [w456 _]
          frame True {
            n244 = invoke class="IICImagingControl" method="LiveStop"(reference=w456) -> ()  [unwired: 2 in, 3 out]
          }
          frame False {
          }
        }
      }
    }
  }
